vi "Write Status.vi"(10 "Status":string, 11 "States In":string) -> (7 "States Out":string)   [LabVIEW 2019]
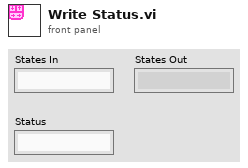
[diagram p1: front panel]
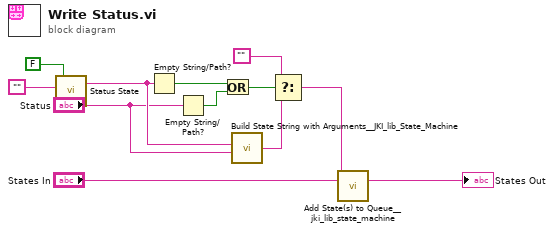
[diagram p0: block diagram]
diagram:
  n1 = call "Status State.vi"("Status State In"="", "Write"=FALSE) -> ("Status State Out"=w12:string)  [unwired: 3 in]
  n2 = Empty String/Path?(string/path=w12) -> (empty?=w9:bool)
  n3 = Empty String/Path?(string/path="Status") -> (empty?=w10:bool)
  n4 = Or(x=w9, y=w10) -> (x .or. y?=w8:bool)
  n5 = call <vilib>:"Build State String with Arguments__JKI_lib_State_Machine.vi"("Arguments (\"\")"="Status", "State"=w12) -> ("State with Arguments"=w7:string)  [unwired: 4 in]
  n6 = Select(t="", s=w8, f=w7) -> (s? t:f=w5:string)
  n7 = call <vilib>:"Add State(s) to Queue__jki_lib_state_machine.vi"("State(s) in Front (\"\")"=w5, "State(s) in (\"\")"="States In") -> ("States Out"=→"States Out":string)  [unwired: 13 in]
